vi "Handle getAll.vi"(8 "error in (no error)":errorcluster, 11 "Inst.RP100 in":refnum<class "Inst.RP100.lvclass">) -> (0 "error out":errorcluster, 2 "getAll":variant, 3 "Inst.RP100 out":refnum<class "Inst.RP100.lvclass">)   [LabVIEW 2019, in "Inst.RP100.lvlib" / "Inst.RP100.lvclass"]
uses:
  Inst.RP100.lvclass
  Inst.RP100.lvclass/Inst.RP100.ctl
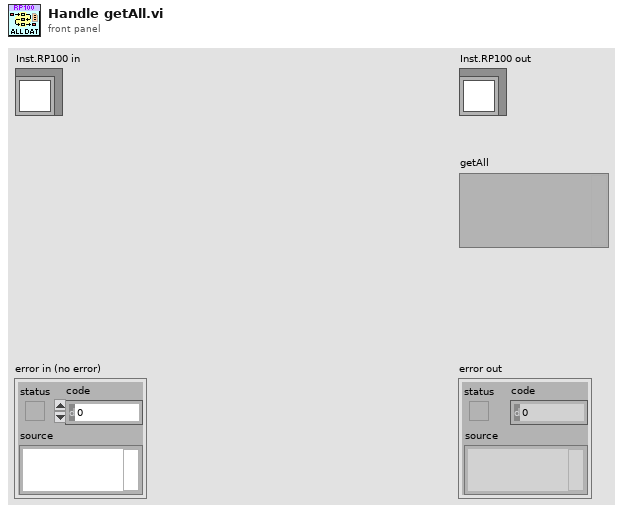
[diagram p1: front panel]
types:
  T1 = typedef "Inst.RP100.lvlib/Inst.RP100.lvclass/Inst.RP100.getAll--Cluster.ctl" = cluster{"OutputStateCh1":string, "OutputStateCh2":string, "LevelCh1":dbl, "LevelCh2":dbl, "SlewCh1":dbl, "SlewCh2":dbl, "MeasuredVCh1":dbl, "MeasuredVCh2":dbl, "MeasuredICh1":dbl, "MeasuredICh2":dbl}
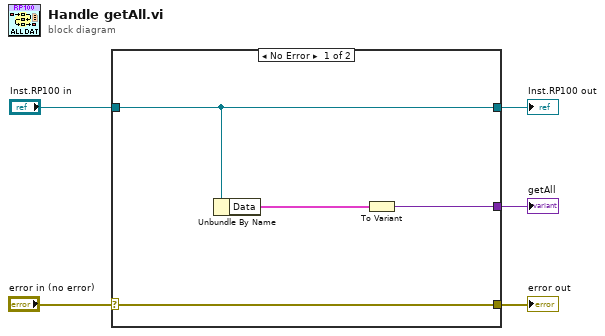
[diagram p0: block diagram]
diagram:
  n1 = case shown="No Error" "error in (no error)" {
    selector: "error in (no error)" -> [w8 w11]
    tunnel: [w8 w11] -> w3
    tunnel: [w6 w10] -> w1
    tunnel: "Inst.RP100 in" -> [w6 w10]
    tunnel: [w9 _] -> w2
    frame No Error {
      n2 = Unbundle By Name(w6) -> ("Data"=w7:T1)
      n3 = To Variant(anything=w7) -> (Variant=w9:variant)
    }
    frame Error {
    }
  }
  "error out" <- w3
  "Inst.RP100 out" <- w1
  "getAll" <- w2
